vi "crossedLineWayPoint.vi"(0 "X Boat (Pixel)":dbl, 1 "Y Boat (Pixel)":dbl, 2 "Current Gate":dbl[](array[numeric])=[200.0, 200.0, 200.0, 800.0], 3 "Past Gate":dbl[](array[numeric])=[500.0, 100.0, 200.0, 200.0], 4 "Boat Heading (Rotated)":dbl) -> (5 "Passed Current Gate?":bool)   [LabVIEW 2012]
panel:
  out "XY Graph":cluster{"X":dbl, "Y":dbl}[](graph)
  out "Y Endpoint 2 (Pixel) 2":dbl
  out "X Endpoint 2 (Pixel) 2":dbl
  out "Y Endpoint 1 (Pixel) 2":dbl
  out "X Endpoint 1 (Pixel) 2":dbl
  out "Y Endpoint 2 (Pixel)":dbl
  out "X Endpoint 2 (Pixel)":dbl
  out "Y Endpoint 1 (Pixel)":dbl
  out "X Endpoint 1 (Pixel)":dbl
  # "Information about the Boat"
  # "Information about the Current Gate"
  # "Information about the Past Gate"
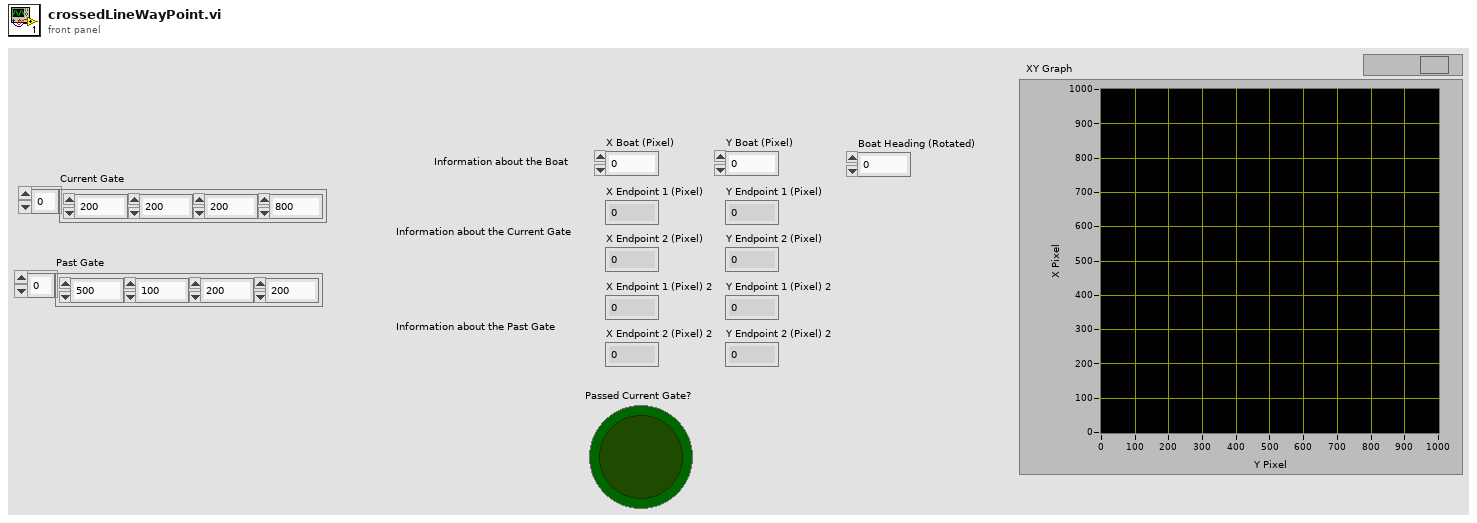
[diagram p1: front panel]
types:
  T1 = cluster{"Y Endpoint 2 (Pixel)":dbl, "X Endpoint 2 (Pixel)":dbl}
  T2 = cluster{"Y Endpoint 1 (Pixel)":dbl, "X Endpoint 1 (Pixel)":dbl}
  T3 = cluster{"Y Boat (Pixel)":dbl, "X Boat (Pixel)":dbl}
  T4 = cluster{"Y Endpoint 1 (Pixel) 2":dbl, "X Endpoint 1 (Pixel) 2":dbl}
  T5 = cluster{"Y Endpoint 2 (Pixel) 2":dbl, "X Endpoint 2 (Pixel) 2":dbl}
  T6 = cluster{"Y Endpoint 2 (Pixel) 2":dbl, "X Endpoint 2 (Pixel) 2":dbl}[]
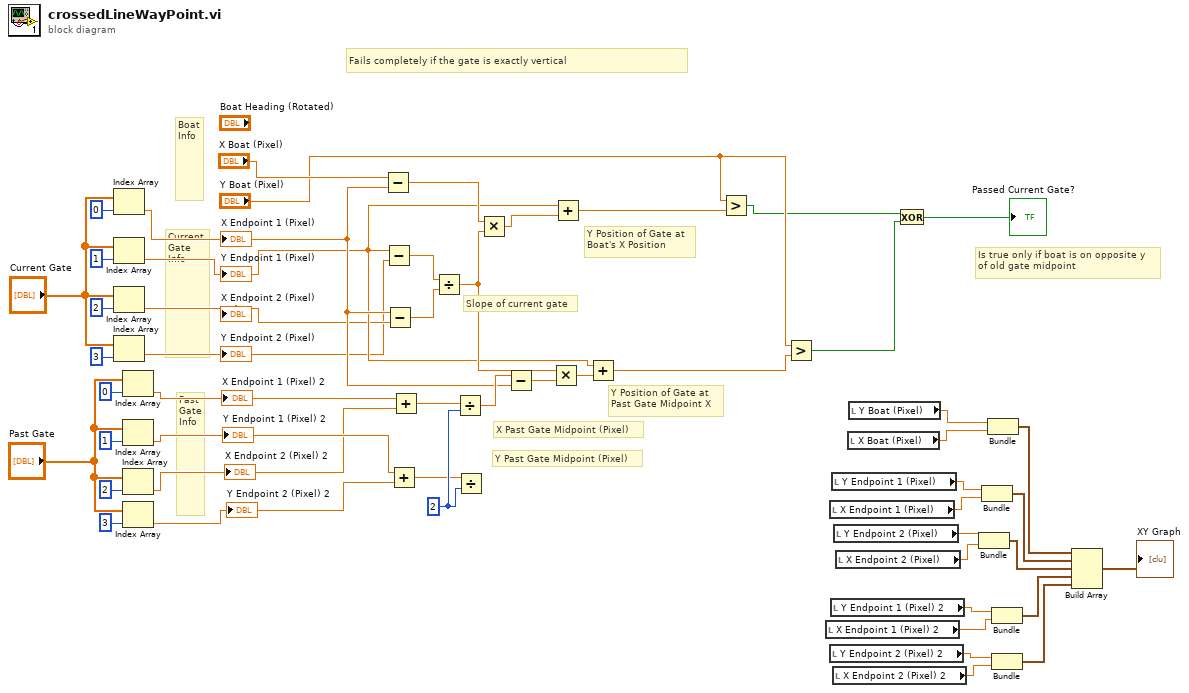
[diagram p0: block diagram]
diagram:
  w52 = 2
  # "Fails completely if the gate is exactly vertical"
  # "Is true only if boat is on opposite y\nof old gate midpoint"
  # "Y Position of Gate at\nPast Gate Midpoint X"
  # "Y Position of Gate at\nBoat's X Position"
  # "Slope of current gate"
  # "Y Past Gate Midpoint (Pixel)"
  # "X Past Gate Midpoint (Pixel)"
  # "Past\nGate\nInfo"
  # "Current\nGate\nInfo"
  # "Boat\nInfo"
  n1 = Index Array(array="Current Gate", index=0) -> (element=w13:dbl)
  "X Endpoint 1 (Pixel)" <- w13
  n2 = Index Array(array="Current Gate", index=1) -> (element=w12:dbl)
  "Y Endpoint 1 (Pixel)" <- w12
  n3 = Index Array(array="Current Gate", index=2) -> (element=w11:dbl)
  "X Endpoint 2 (Pixel)" <- w11
  n4 = Index Array(array="Current Gate", index=3) -> (element=w10:dbl)
  "Y Endpoint 2 (Pixel)" <- w10
  n5 = Index Array(array="Past Gate", index=0) -> (element=w4:dbl)
  "X Endpoint 1 (Pixel) 2" <- w4
  n6 = Index Array(array="Past Gate", index=1) -> (element=w3:dbl)
  "Y Endpoint 1 (Pixel) 2" <- w3
  n7 = Index Array(array="Past Gate", index=2) -> (element=w2:dbl)
  "X Endpoint 2 (Pixel) 2" <- w2
  n8 = Index Array(array="Past Gate", index=3) -> (element=w1:dbl)
  "Y Endpoint 2 (Pixel) 2" <- w1
  n9 = Subtract(x="X Boat (Pixel)", y=w13) -> (x-y=w46:dbl)
  n10 = Subtract(x=w12, y=w10) -> (x-y=w49:dbl)
  n11 = Subtract(x=w13, y=w11) -> (x-y=w48:dbl)
  n12 = Add(x=w3, y=w1) -> (x+y=w51:dbl)
  n13 = Add(x=w4, y=w2) -> (x+y=w50:dbl)
  n14 = Divide(x=w49, y=w48) -> (x/y=w42:dbl)
  n15 = Divide(x=w50, y=w52) -> (x/y=w44:dbl)
  n16 = Divide(x=w51, y=w52) -> ()  [unwired: 1 out]
  n17 = Multiply(x=w46, y=w42) -> (x*y=w45:dbl)
  n18 = Subtract(x=w44, y=w13) -> (x-y=w43:dbl)
  n19 = Multiply(x=w42, y=w43) -> (x*y=w41:dbl)
  n20 = Add(x=w12, y=w45) -> (x+y=w39:dbl)
  n21 = Add(x=w12, y=w41) -> (x+y=w40:dbl)
  n22 = Greater?(x="Y Boat (Pixel)", y=w39) -> (0:w37:bool)
  n23 = Greater?(x="Y Boat (Pixel)", y=w40) -> (0:w36:bool)
  n24 = local read "X Endpoint 1 (Pixel) 2"() -> (w23:dbl)
  n25 = local read "X Endpoint 1 (Pixel)"() -> (w29:dbl)
  n26 = local read "Y Endpoint 2 (Pixel) 2"() -> (w21:dbl)
  n27 = local read "Y Endpoint 1 (Pixel) 2"() -> (w24:dbl)
  n28 = local read "Y Endpoint 1 (Pixel)"() -> (w30:dbl)
  n29 = local read "X Endpoint 2 (Pixel) 2"() -> (w20:dbl)
  n30 = local read "Y Endpoint 2 (Pixel)"() -> (w27:dbl)
  n31 = local read "X Endpoint 2 (Pixel)"() -> (w26:dbl)
  n32 = local read "X Boat (Pixel)"() -> (w33:dbl)
  n33 = local read "Y Boat (Pixel)"() -> (w34:dbl)
  n34 = Exclusive Or(1:w36, 2:w37) -> (0:→"Passed Current Gate?":bool)
  n35 = Bundle("Y Endpoint 2 (Pixel)"=w27, "X Endpoint 2 (Pixel)"=w26) -> (w25:T1)  [unwired: 1 in]
  n36 = Bundle("Y Endpoint 1 (Pixel)"=w30, "X Endpoint 1 (Pixel)"=w29) -> (w28:T2)  [unwired: 1 in]
  n37 = Bundle("Y Boat (Pixel)"=w34, "X Boat (Pixel)"=w33) -> (w32:T3)  [unwired: 1 in]
  n38 = Bundle("Y Endpoint 1 (Pixel) 2"=w24, "X Endpoint 1 (Pixel) 2"=w23) -> (w22:T4)  [unwired: 1 in]
  n39 = Bundle("Y Endpoint 2 (Pixel) 2"=w21, "X Endpoint 2 (Pixel) 2"=w20) -> (w19:T5)  [unwired: 1 in]
  n40 = Build Array(w32, w28, w25, w22, w19) -> (→"XY Graph":T6)
